vi "Set Voltage Dither via Desired Filtered Moisture.vi"(8 "Error In":errorcluster, 11 "Desired FilteredMoisture":dbl=2400.0 min=1000.0 max=6300.0 step=5.0) -> (0 "Error Out":errorcluster)   [LabVIEW 2016]
uses:
  Tools/Laundry/JL Dryer Tool/JL Dryer Tool Support/UTL_JL Scaling Factor Folder/Controls/ENUM_JL Scaling Factor_.ctl
  DAQ/Controls/Moisture Data.ctl
panel:
  out "Analog Value Out":dbl
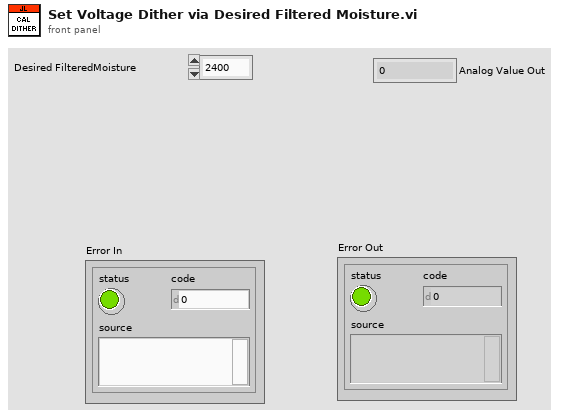
[diagram p1: front panel]
types:
  T1 = cluster{"Calibrate?":bool, "Scalling In ":cluster{"Raw Low ":dbl, "Raw High":dbl, "Actual Low":dbl, "Actual High":dbl}}
  T2 = cluster{"Raw Low ":dbl, "Raw High":dbl, "Actual Low":dbl, "Actual High":dbl}
  T3 = typedef "Moisture Data.ctl" = cluster{"Moisture (V)":dbl, "Dither":dbl, "Stop":bool}
  T4 = typedef "ENUM_JL Scaling Factor_.ctl" = enum16{"Init", "Scale Voltage", "Flush Slope"}
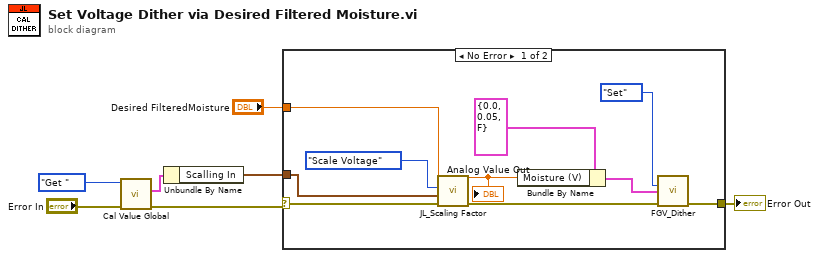
[diagram p0: block diagram]
diagram:
  n1 = call "Cal Value Global.vi"("error in (no error)"="Error In", "Action"=enum16{"Set", "Get "}."Get ") -> ("error out"=w1:errorcluster, "Cal  Out"=w4:T1)  [unwired: 8 in]
  n2 = Unbundle By Name(w4) -> ("Scalling In"=w3:T2)
  n3 = case shown="No Error" w1 {
    selector: w1 -> [w9 w18]
    tunnel: "Desired FilteredMoisture" -> [w17 _]
    tunnel: [w10 w18] -> w7
    tunnel: w3 -> [w8 _]
    frame No Error {
      n4 = call "JL_Scaling Factor.vi"("Error"=w9, "Scalling"=w8, "Scaling Type"=ENUM_JL_Scaling_Factor_."Scale Voltage", "Desired Value Out"=w17) -> ("Error Out"=w11:errorcluster, "Analog Value Out"=w14:dbl)  [unwired: 5 in, 1 out]
      "Analog Value Out" <- w14
      n5 = Bundle By Name(cluster=T3 {"Moisture (V)"=0.0, "Dither"=0.05, "Stop"=FALSE} ("Moisture Data In"), "Moisture (V)"=w14) -> (w13:T3)
      n6 = call "FGV_Dither.vi"("Action"=enum16{"Set", "Get "}."Set", "Moisture Data In"=w13, "Error In"=w11) -> ("Error Out"=w10:errorcluster)  [unwired: 11 in, 1 out]
    }
    frame Error {
    }
  }
  "Error Out" <- w7
